vi "Message Forward Out.vi"(8 "error in (no error)":errorcluster, 10 "Node Actor MSG In":refnum<class "Node Actor MSG.lvclass">, 11 "Node Actor in":refnum<class "Node Actor.lvclass">) -> (0 "error out":errorcluster, 3 "Node Actor out":refnum<class "Node Actor.lvclass">)   [LabVIEW 2024, in "Node Actor.lvclass"]
uses:
  Node Actor.lvclass
  Node Actor MSG/Node Actor MSG.lvclass
  Node Actor MSG/Node Actor MSG.lvclass/Node Actor MSG.ctl
  Node Actor.lvclass/Node Actor.ctl
  Node Actor MSG/Public Data/Read Forward ID.vi
  Node Actor MSG/Public Data/Read Forward Message.vi
  Node Actor MSG/Public Data/Read Forward Tag.vi
  Node Actor MSG/Public Data/Read Message Forward Target Type.vi
  Message/Message.lvclass
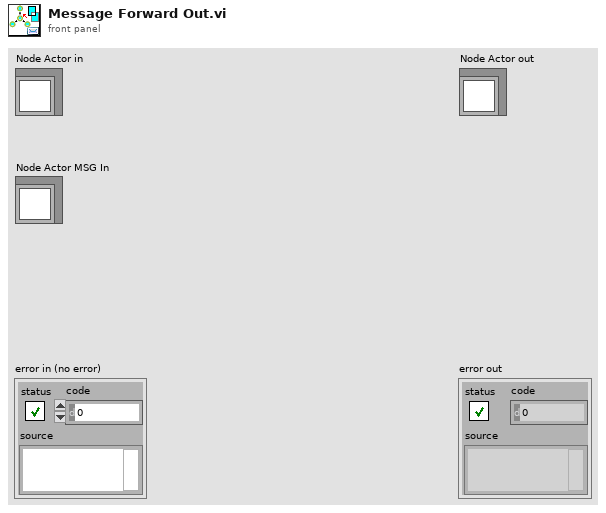
[diagram p1: front panel]
types:
  T1 = typedef "Message Forward Target Type.ctl" = enum16{"None", "ID", "Tag", "Mail Startegy", "Task"}
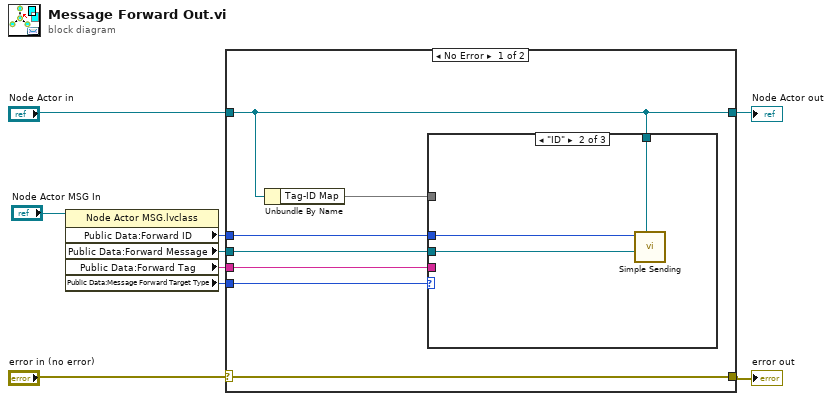
[diagram p0: block diagram]
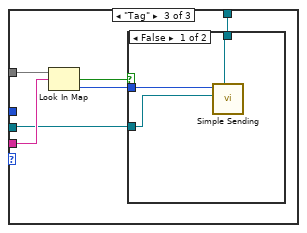
[diagram p3: hidden frame]
diagram:
  n1 = property class="Node Actor MSG.lvclass"(reference="Node Actor MSG In") -> ("Public Data:Forward ID"=w8:i64, "Public Data:Forward Message"=w7:refnum<class "Message.lvclass">, "Public Data:Forward Tag"=w6:string, "Public Data:Message Forward Target Type"=w9:T1)  [unwired: 1 in, 2 out]
  n2 = case shown="No Error" "error in (no error)" {
    selector: "error in (no error)" -> [w16 w30]
    tunnel: [w16 w30] -> w2
    tunnel: [w11 w29] -> w1
    tunnel: "Node Actor in" -> [w11 w29]
    tunnel: w9 -> [w15 _]
    tunnel: w8 -> [w14 _]
    tunnel: w7 -> [w13 _]
    tunnel: w6 -> [w12 _]
    frame No Error {
      n3 = Unbundle By Name(w11) -> ("Tag-ID Map"=w10:map{string, i64})
      n4 = case shown="\"ID\"" w15 {
        tunnel: w14 -> [_ w18 _]
        tunnel: w13 -> [_ w17 w20]
        tunnel: w12 -> [_ _ w24]
        tunnel: w11 -> [_ w19 w22]
        tunnel: w10 -> [_ _ w25]
        frame "None", Default {
        }
        frame "ID" {
          n5 = call "Simple Sending.vi"("System Actor In"=w19, "Message In"=w17, "ID In"=w18) -> ()  [unwired: 9 in]
        }
        frame "Tag" {
          n6 = Look In Map(map=w25, key=w24) -> (key not found?=w23:bool, value=w21:i64)  [unwired: 1 in]
          n7 = case shown="False" w23 {
            tunnel: w22 -> [w28 _]
            tunnel: w21 -> [w27 _]
            tunnel: w20 -> [w26 _]
            frame False {
              n8 = call "Simple Sending.vi"("System Actor In"=w28, "Message In"=w26, "ID In"=w27) -> ()  [unwired: 9 in]
            }
            frame True {
            }
          }
        }
      }
    }
    frame Error {
    }
  }
  "error out" <- w2
  "Node Actor out" <- w1
